vi "Add Memory Channels.vi"(8 "error in (no error)":errorcluster, 11 "Item Ref in":T1 format="%.0x") -> (0 "error out":errorcluster, 3 "Item Ref out":T1 format="%.0x")   [LabVIEW 2027, in "System Monitor System Explorer.lvlib"]
uses:
  System Monitor System Explorer.lvlib
  <vilib>/NI VeriStand/Custom Device API/Custom Device Item Ref.ctl
  <vilib>/NI VeriStand/Custom Device API/Custom Device Channel.ctl
  <vilib>/NI VeriStand/Custom Device API/Custom Device Channel Type.ctl
  <vilib>/NI VeriStand/Custom Device API/Custom Device API.lvlib
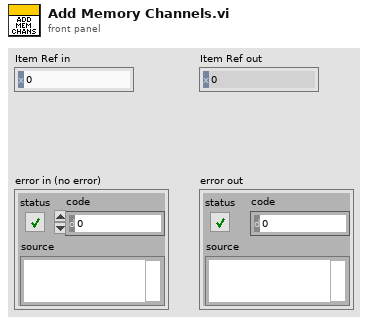
[diagram p1: front panel]
types:
  T1 = typedef "Custom Device API.lvlib/Custom Device Item Ref.ctl" = u64
  T2 = typedef "Custom Device API.lvlib/Custom Device Channel.ctl" = cluster{"Type":T3, "Units":string, "Default Value":dbl, "Faultable":bool, "Scalable":bool}
  T3 = typedef "Custom Device API.lvlib/Custom Device Channel Type.ctl" = enum16{"Input", "Output"}
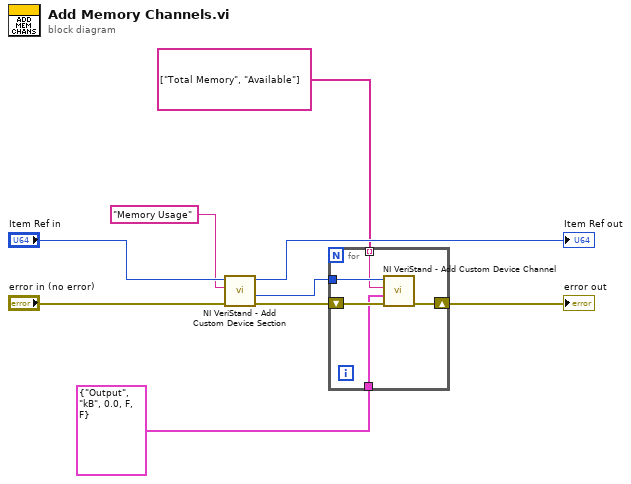
[diagram p0: block diagram]
diagram:
  n1 = call <vilib>:"NI VeriStand - Add Custom Device Section.vi"("error in (no error)"="error in (no error)", "Section Name"="Memory Usage", "Parent Ref in"="Item Ref in") -> ("error out"=w6:errorcluster, "Section Ptr"=w5:T1, "Parent Ref out"=→"Item Ref out":T1)  [unwired: 5 in, 1 out]
  n2 = for {
    tunnel: w5 -> [w13]
    shift-right: [w12] -> w3
    shift-left: w6 -> [w14]
    tunnel: string[] ["Total Memory", "Available"] -> [w11] mode=indexing
    tunnel: T2 {"Type"=enum."Output", "Units"="kB", "Default Value"=0.0, "Faultable"=FALSE, "Scalable"=FALSE} ("Channel") -> [w10]
    n3 = call <vilib>:"NI VeriStand - Add Custom Device Channel.vi"("error in (no error)"=w14, "Channel"=w10, "Channel Name"=w11, "Parent Ref in"=w13) -> ("error out"=w12:errorcluster)  [unwired: 4 in, 3 out]
  }
  "error out" <- w3
